vi "closeXMLFile.vi"(8 "error in (no error)":errorcluster, 11 "XmlParser in":refnum<class "XmlParser.lvclass">) -> (0 "error out":errorcluster, 3 "XmlParser out":refnum<class "XmlParser.lvclass">)   [LabVIEW 2009, in "Tools.lvlib" / "xml.lvlib" / "XmlParser.lvclass"]
doc: "Close the xml document so others can use it."
uses:
  XmlParser.lvclass
  XmlParser.lvclass/XmlParser.ctl
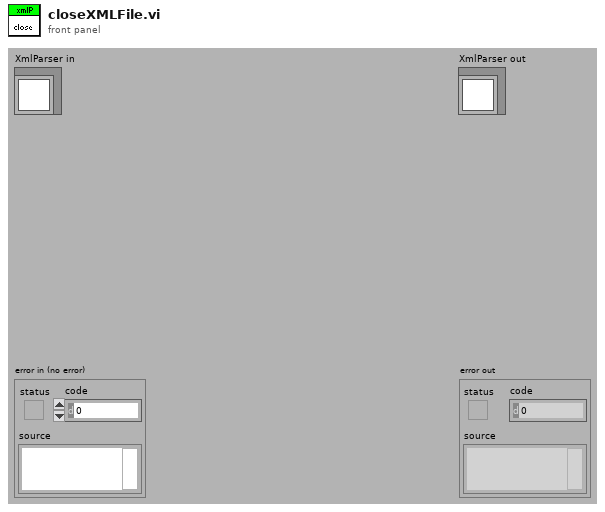
[diagram p1: front panel]
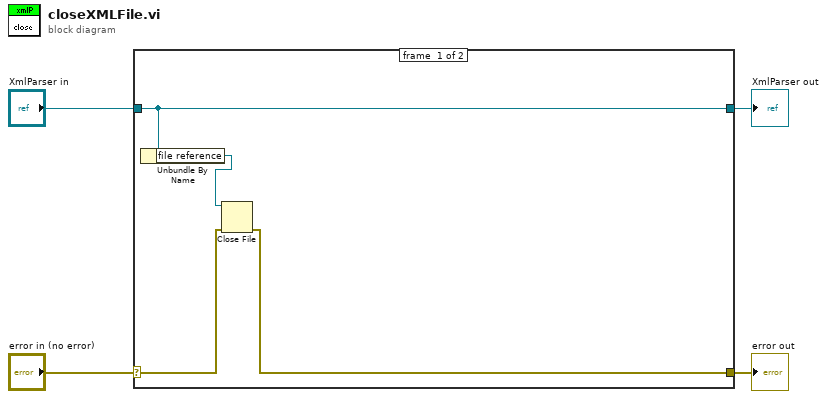
[diagram p0: block diagram]
diagram:
  n1 = case shown="No Error" "error in (no error)" {
    selector: "error in (no error)" -> [w8 w10]
    tunnel: [w7 w10] -> w3
    tunnel: [w6 w9] -> w1
    tunnel: "XmlParser in" -> [w6 w9]
    frame #0 {
      n2 = Unbundle By Name(w6) -> ("file reference"=w5:refnum<file>)
      n3 = Close File(refnum=w5, error in=w8) -> (error out=w7:errorcluster)  [unwired: 1 out]
    }
    frame #1 {
    }
  }
  "error out" <- w3
  "XmlParser out" <- w1
